vi "MGI Set Logging Parameters.vi"(9 "Max # Log Files (Don't change)":i32=-2, 10 "Max # Errors to Log (Don't change)":i32=-2, 11 "MGI Error Reporter Base In":refnum<class "MGI Error Reporter Base.lvclass">) -> (3 "MGI Error Reporter Base Out":refnum<class "MGI Error Reporter Base.lvclass">)   [LabVIEW 2020, in "MGI Error Reporter Base.lvclass"]
doc: "Sets the behavior of the Error Logger. Default behavior is to log a maximum of 5000 errors per file and to keep a maximum of 100 files.\nMax # Errors to Log is the number of errors logged to a file where subsequent errors are not logged. Wire a -2 to leave this number unchanged. Wire a -1 to log all errors to file. Wire a 0 to disable error logging.\nMax # Log Files is the number of error logs in the error directory. The oldest log files are deleted to make room for new files. Wire -2 to leave this number unchanged. Wire a -1 to disable the deletion of older files. Wire a 0 to disable error logging.\n\n\nAuthored by Shawn Walpole\nsupport@mooregoodideas.com\nwww.mooregoodideas.com\n\nCopyright (c) 2010, Moore Good Ideas, Inc.\n\nAll rights reserved.\n\nRedistribution and use in source and binary forms, with or without modification, are permitted provided that the following conditions are met:\n\n * Redistributions of source code must retain the above copyright notice, this list of conditions and the following disclaimer.\n * Redistributions in binary form must reproduce the above copyright notice, this list of conditions and the following disclaimer in the documentation and/or other materials provided with the distribution.\n * Neither the name of Moore Good Ideas, Inc. nor the names of its contributors may be used to endorse or promote products derived from this software without specific prior written permission.\n\nTHIS SOFTWARE IS PROVIDED BY THE COPYRIGHT HOLDERS AND CONTRIBUTORS \"AS IS\" AND ANY EXPRESS OR IMPLIED WARRANTIES, INCLUDING, BUT NOT LIMITED TO, THE IMPLIED WARRANTIES OF MERCHANTABILITY AND FITNESS FOR A PARTICULAR PURPOSE ARE DISCLAIMED. IN NO EVENT SHALL THE COPYRIGHT OWNER OR CONTRIBUTORS BE LIABLE FOR ANY DIRECT, INDIRECT, INCIDENTAL, SPECIAL, EXEMPLARY, OR CONSEQUENTIAL DAMAGES (INCLUDING, BUT NOT LIMITED TO, PROCUREMENT OF SUBSTITUTE GOODS OR SERVICES; LOSS OF USE, DATA, OR PROFITS; OR BUSINESS INTERRUPTION) HOWEVER CAUSED AND ON ANY THEORY OF LIABILITY, WHETHER IN CONTRACT, STRICT LIABILITY, OR TORT (INCLUDING NEGLIGENCE OR OTHERWISE) ARISING IN ANY WAY OUT OF THE USE OF THIS SOFTWARE, EVEN IF ADVISED OF THE POSSIBILITY OF SUCH DAMAGE."
uses:
  <userlib>/_MGI/Error Reporter/MGI Error Reporter Base/MGI Error Reporter Base.lvclass
  <userlib>/_MGI/Error Reporter/MGI Error Reporter Base/MGI Error Reporter Base.lvclass/MGI Error Reporter Base.ctl
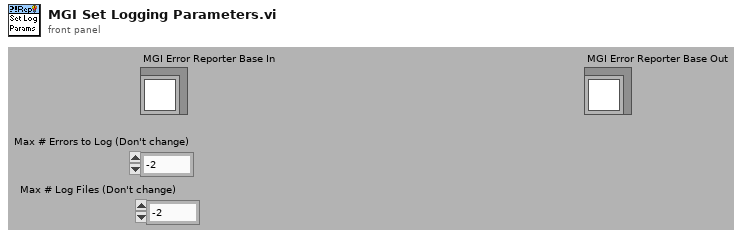
[diagram p1: front panel]
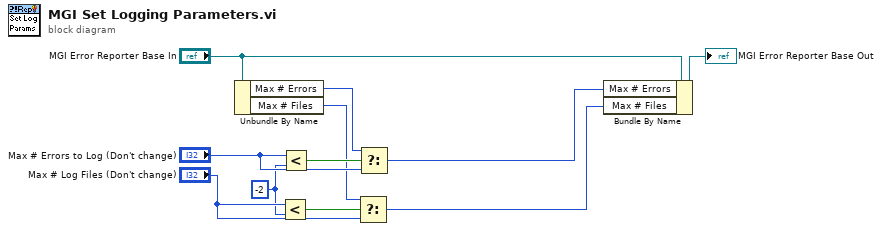
[diagram p0: block diagram]
diagram:
  w2 = -2 ("y")
  n1 = Unbundle By Name("MGI Error Reporter Base In") -> ("Max # Errors"=w8:i32, "Max # Files"=w3:i32)
  n2 = Less?(x="Max # Log Files (Don't change)", y=w2) -> (x < y?=w5:bool)
  n3 = Less?(x="Max # Errors to Log (Don't change)", y=w2) -> (x < y?=w9:bool)
  n4 = Select(t=w3, s=w5, f="Max # Log Files (Don't change)") -> (s? t:f=w1:i32)
  n5 = Select(t=w8, s=w9, f="Max # Errors to Log (Don't change)") -> (s? t:f=w7:i32)
  n6 = Bundle By Name(cluster="MGI Error Reporter Base In", "Max # Errors"=w7, "Max # Files"=w1) -> (→"MGI Error Reporter Base Out":refnum<class "MGI Error Reporter Base.lvclass">)
